vi "Update Flow.vi"(8 "error in (no error)":errorcluster, 11 "Flow":dbl) -> (0 "error out":errorcluster)   [LabVIEW 2015, in "Model.lvlib"]
uses:
  Model.lvlib
  Solution/Production Line/support/Message Queue/Message Queue.lvlib
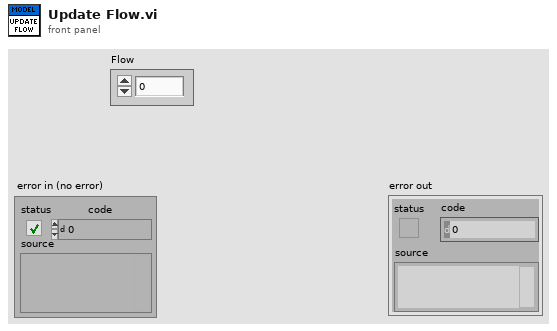
[diagram p1: front panel]
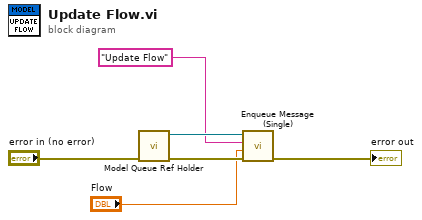
[diagram p0: block diagram]
diagram:
  n1 = call "Model Queue Ref Holder.vi"("error in"="error in (no error)") -> ("error out"=w6:errorcluster, "Input Message Queue"=w3:refnum<queue>)  [unwired: 9 in]
  n2 = call "Enqueue Message (Single).vi"("error in (no error)"=w6, "Message Data"="Flow", "Message"="Update Flow", "Message Queue"=w3) -> ("error out"=→"error out":errorcluster)  [unwired: 6 in, 1 out]
